vi "Estimate total time.vi"(8 "error in (no error)":errorcluster, 11 "Tomo in":refnum<class "Tomo.lvclass">) -> (0 "error out":errorcluster, 3 "Tomo out":refnum<class "Tomo.lvclass">)   [LabVIEW 2012, in "Tomo.lvclass"]
uses:
  Tomo.lvclass
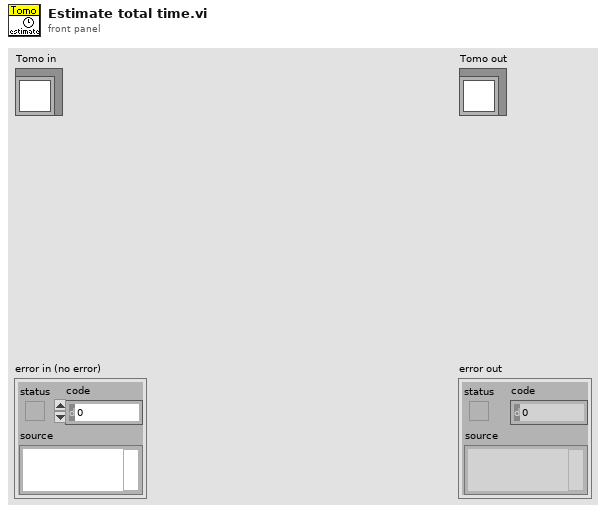
[diagram p1: front panel]
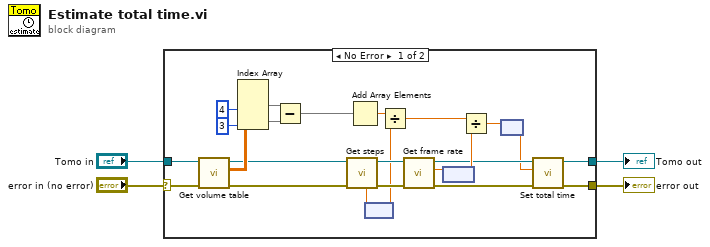
[diagram p0: block diagram]
diagram:
  n1 = case shown="No Error" "error in (no error)" {
    selector: "error in (no error)" -> [w28 w30]
    tunnel: [w10 w30] -> w3
    tunnel: [w8 w29] -> w1
    tunnel: "Tomo in" -> [w27 w29]
    frame No Error {
      n2 = call-dynamic "Get volume table.vi"("error in (no error)"=w28, "Tomo in"=w27) -> ("error out"=w21:errorcluster, "Volume table out"=w26:dbl[][], "Tomo out"=w19:refnum<class "Tomo.lvclass">)  [unwired: 7 in]
      n3 = Index Array(array=w26, index (col) #1=4 ("disabled index (col)"), index (col) #2=3 ("index (col)")) -> (element #1=w23:dbl[], element #2=w22:dbl[])  [unwired: 2 in]
      n4 = Subtract(x=w23, y=w22) -> (x-y=w5:dbl[])
      n5 = call-dynamic "Get steps.vi"("error in (no error)"=w21, "Tomo in"=w19) -> ("error out"=w20:errorcluster, "Tomo out"=w18:refnum<class "Tomo.lvclass">, "Z step size"=w16:dbl[unit])  [unwired: 4 in, 3 out]
      n6 = Add Array Elements(numeric array=w5) -> (sum=w17:dbl)
      n7 = node(w16) -> (w13:dbl)
      n8 = Divide(x=w17, y=w13) -> (x/y=w14:dbl)
      n9 = call-dynamic "Get frame rate.vi"("error in (no error)"=w20, "Tomo in"=w18) -> ("error out"=w11:errorcluster, "Frame rate"=w15:dbl[unit], "Tomo out"=w9:refnum<class "Tomo.lvclass">)  [unwired: 7 in]
      n10 = node(w15) -> (w12:dbl)
      n11 = Divide(x=w14, y=w12) -> (x/y=w6:dbl)
      n12 = node(w6) -> (w7:dbl[unit])
      n13 = call-dynamic "Set total time.vi"("error in (no error)"=w11, "Total time"=w7, "Tomo in"=w9) -> ("error out"=w10:errorcluster, "Tomo out"=w8:refnum<class "Tomo.lvclass">)  [unwired: 7 in]
    }
    frame Error {
    }
  }
  "error out" <- w3
  "Tomo out" <- w1
